vi "Decorate.vi"(8 "error in (no error)":errorcluster, 10 "Beverage.lvclass":refnum<class "Beverage.lvclass">, 11 "Soy in":refnum<class "Soy.lvclass">) -> (0 "error out":errorcluster, 3 "Soy out":refnum<class "Soy.lvclass">)   [LabVIEW 2013, in "Soy.lvclass"]
uses:
  Soy.lvclass
  Beverage/Beverage.lvclass
  Soy.lvclass/Soy.ctl
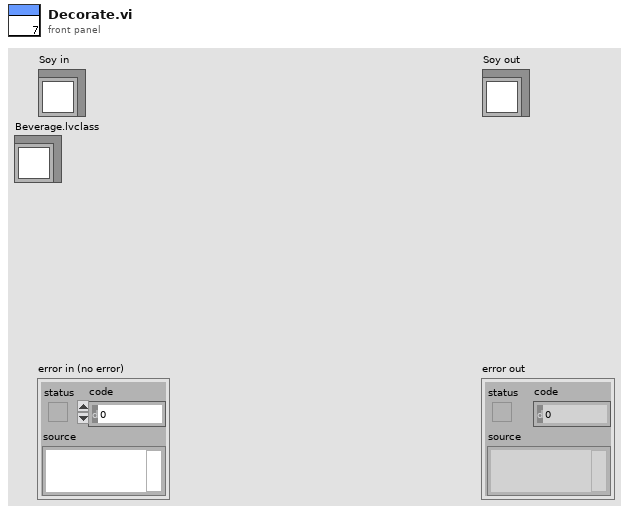
[diagram p1: front panel]
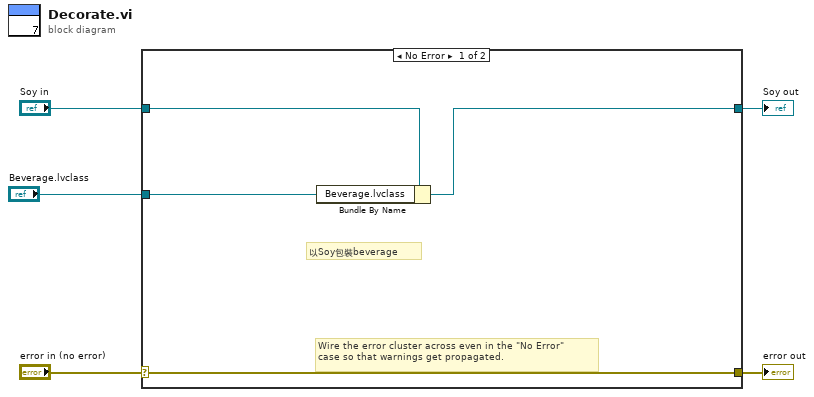
[diagram p0: block diagram]
diagram:
  n1 = case shown="No Error" "error in (no error)" {
    selector: "error in (no error)" -> [w9 w11]
    tunnel: [w9 w11] -> w4
    tunnel: [w7 w10] -> w2
    tunnel: "Soy in" -> [w8 w10]
    tunnel: "Beverage.lvclass" -> [w6 _]
    frame No Error {
      # "以Soy包裝beverage"
      # "Wire the error cluster across even in the \"No Error\"\ncase so that warnings get propagated."
      n2 = Bundle By Name(cluster=w8, "Beverage.lvclass"=w6) -> (w7:refnum<class "Soy.lvclass">)
    }
    frame Error {
    }
  }
  "error out" <- w4
  "Soy out" <- w2
